vi "Gas-control-ideas.vi"() -> ()   [LabVIEW 2021]
panel:
  out "Time has Elapsed":bool
  out "Elapsed Time (s)":dbl format="%.1f"
  in  "ENA":bool
  in  "Automatic":bool
  out "Boolean":bool
  in  "Power Button":bool
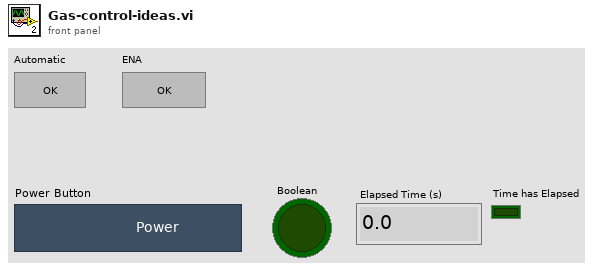
[diagram p1: front panel]
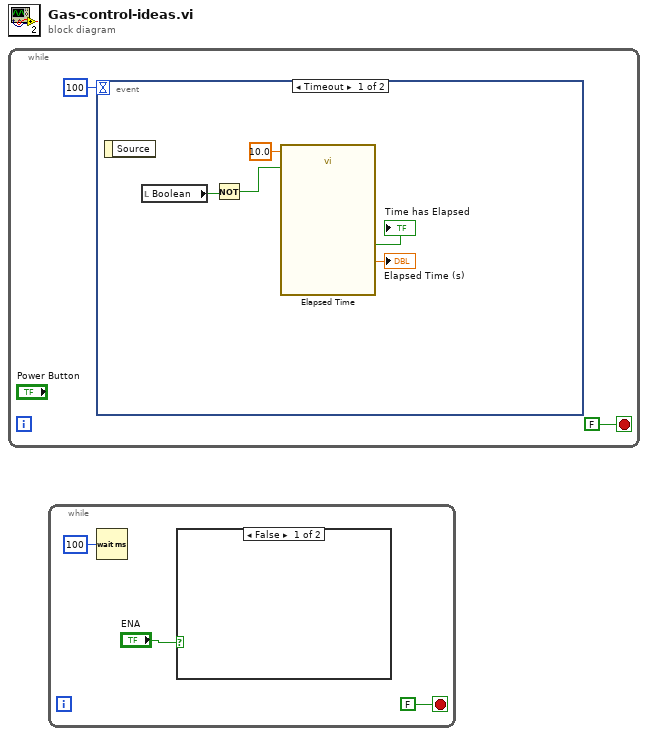
[diagram p0: block diagram]
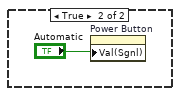
[diagram p2: hidden frame]
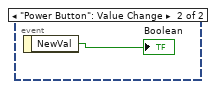
[diagram p3: hidden frame]
diagram:
  n1 = while {
    stop <- FALSE stop-if-true
    n2 = event shown="[0] Timeout" {
      selector: _ -> [_ _]
      dyn-events: _ -> [_ _]
      timeout: 100 -> [_ _]
      event Timeout {
        n3 = event-data() -> ()  [unwired: 1 in, 1 out]
        n4 = local read "Boolean"() -> (w6:bool)
        n5 = Not(x=w6) -> (.not. x?=w7:bool)
        n6 = call "Elapsed Time"("Time Target (s)"=10.0, "Reset"=w7) -> ("Elapsed Time (s)"=→"Elapsed Time (s)":dbl, "Time has Elapsed"=→"Time has Elapsed":bool)  [unwired: 10 in, 6 out]
      }
      event "Power Button": Value Change {
        n7 = event-data() -> ("NewVal"=→"Boolean":bool)  [unwired: 1 in]
      }
    }
  }
  n8 = while {
    stop <- FALSE stop-if-true
    n9 = Wait (ms)(milliseconds to wait=u32 100) -> ()  [unwired: 1 out]
    n10 = case shown="False" "ENA" {
      frame False {
      }
      frame True {
        n11 = property on="Power Button" class="Bool (strict)"("Val(Sgnl)"="Automatic") -> ()  [unwired: 2 in, 2 out]
      }
    }
  }
